vi "Remove.vi"(11 "TypedCircularBuffer in":refnum<class "VarCircularBuffer.lvclass">) -> (1 "invalid?":bool, 2 "element":variant=variant(i32 0), 3 "TypedCircularBuffer out":refnum<class "VarCircularBuffer.lvclass">)   [LabVIEW 2024, in "VarCircularBuffer.lvclass"]
uses:
  VarCircularBuffer.lvclass
  VarCircularBuffer.lvclass/VarCircularBuffer.ctl
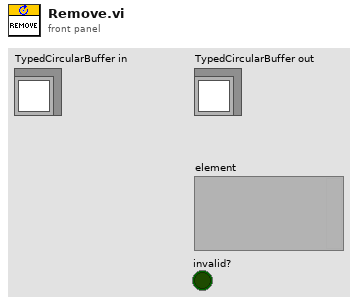
[diagram p1: front panel]
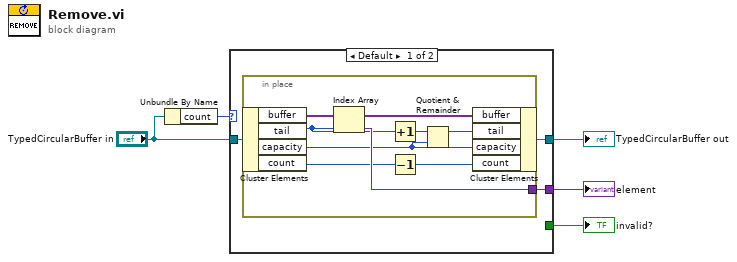
[diagram p0: block diagram]
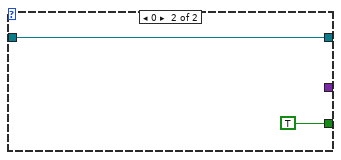
[diagram p2: hidden frame]
diagram:
  n1 = Unbundle By Name("TypedCircularBuffer in") -> ("count"=w2:u32)
  n2 = case shown="Default" w2 {
    tunnel: "TypedCircularBuffer in" -> [w8 w18]
    tunnel: [w7 _] -> w3
    tunnel: [w6 w18] -> w4
    tunnel: [_ TRUE] -> w1
    frame Default {
      n3 = in-place {
        in-place-border: [w16] -> w7
        n4 = in-place-cluster #1(w8) -> ("buffer"=w9:variant[], "tail"=w13:u32, "capacity"=w10:u32, "count"=w15:u32)
        n5 = Index Array(array=w9, index=w13) -> (element=w16:variant)
        n6 = Increment(x=w13) -> (x+1=w12:u32)
        n7 = Decrement(x=w15) -> (x-1=w14:u32)
        n8 = Quotient & Remainder(x=w12, y=w10) -> (x-y*floor(x/y)=w11:u32)  [unwired: 1 out]
        n9 = in-place-cluster #1("buffer"=w9, "tail"=w11, "capacity"=w10, "count"=w14) -> (w6:refnum<class "VarCircularBuffer.lvclass">)
      }
    }
    frame 0 {
    }
  }
  "TypedCircularBuffer out" <- w4
  "element" <- w3
  "invalid?" <- w1
